vi "Initialize.vi"   [LabVIEW 2011, in "Hokuyo URG Series.lvlib"]
doc: "Establishes communication with the instrument. It also places the instrument in a default state needed for other instrument driver operations. Therefore, call this VI before calling other instrument driver VIs for this instrument. Generally, you need to call the Initialize VI only once at the beginning of an application."
uses:
  Hokuyo URG Series.lvlib
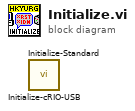
[diagram p0: block diagram]
diagram:
  n1 = call "Initialize-cRIO-USB.vi"() -> ()  [unwired: 10 in, 2 out]
  n2 = call "Initialize-Standard.vi"() -> ()  [unwired: 10 in, 2 out]
